vi "Hasp.vi"(0 "param1":i32, 1 "Service":u16(ring)=8 items=["LocalHasp_IsHasp"=1, "LocalHasp_HaspCode"=2, "LocalHast_ReadWord"=3, "LocalHast_WriteWord"=4, "LocalHasp_HaspStatus/API_Version"=5, "LocalHasp_HaspGeneration"=8, "LocalHasp_HaspNetStatus"=9, "LocalHasp_ReadBlock"=50, "LocalHasp_WriteBlock"=0, "LocalHasp_EncodeData"=60, "LocalHasp_DecodeData"=61, "NEtHasp_EncodeData"=88, "NetHasp_DecodeData"=89], 2 "pass1":i32=15417, 3 "pass2":i32=9632, 5 "param2":i32, 7 "param3":i32=-255 format="%.2f", 9 "param4":i32, 11 "error in (no error)":errorcluster, 12 "lptnum":i32) -> (4 "param1":i32, 6 "param2":i32, 8 "param3":i32=-12, 10 "param4":i32, 15 "error out":errorcluster)   [LabVIEW 2017]
uses:
  Common/Hasp/haspms32.dll
panel:
  in  "seed":i32
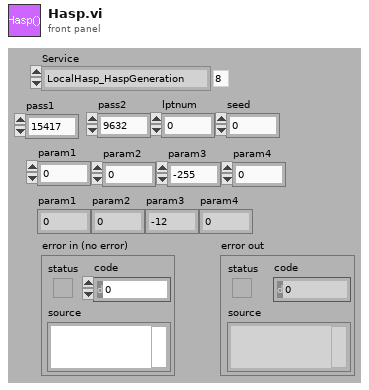
[diagram p1: front panel]
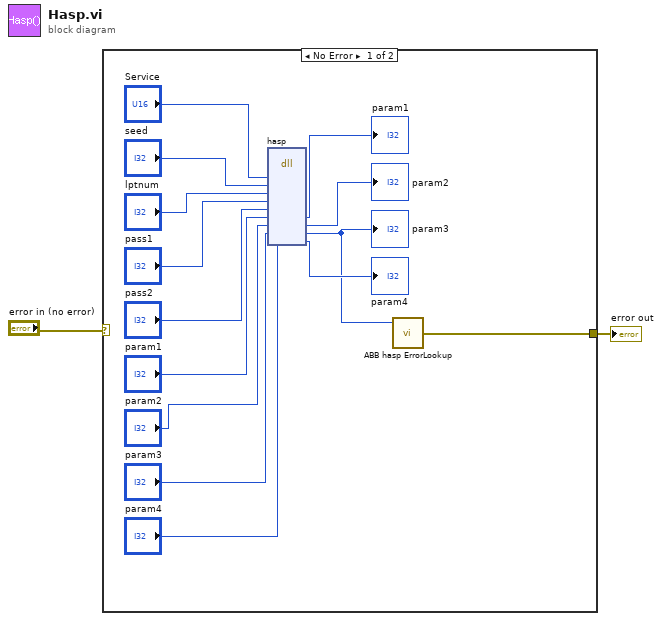
[diagram p0: block diagram]
diagram:
  n1 = case shown="No Error" "error in (no error)" {
    selector: "error in (no error)" -> [_ w17]
    tunnel: [w3 w17] -> w1
    frame No Error {
      n2 = dll-call lib="C:/Projects/Labview Projects/LabView2017/Common/Hasp/haspms32.dll" fn="hasp"("service"="Service", "seed"="seed", "lptnum"="lptnum", "pass1"="pass1", "pass2"="pass2", "param1"="param1", "param2"="param2", "param3"="param3", "param4"="param4") -> ("param1"=→"param1":i32, "param2"=→"param2":i32, "param3"=w4:i32, "param4"=→"param4":i32)  [unwired: 9 in, 2 out]
      "param3" <- w4
      n3 = call "ABB hasp ErrorLookup.vi"("ReturnVal"=w4) -> ("error out"=w3:errorcluster)  [unwired: 2 in]
    }
    frame Error {
    }
  }
  "error out" <- w1
